vi "Get Targets.vi"(7 "Load Stored Targets?(T)":bool=TRUE, 8 "error in (no error)":errorcluster, 11 "Dependency Source in":refnum<class "Dependency Source.lvclass">) -> (0 "error out":errorcluster, 1 "Success?":bool, 2 "External Targets":T3, 3 "Internal Targets":T2, 4 "Unhandled Targets":T1, 5 "Valid Dependency Source?":bool)   [LabVIEW 2019, in "Project.Dependencies Finder.lvlib" / "Dependency Source.lvclass"]
doc: "Get internal and external targets for the dependency source."
uses:
  Dependency Source.lvclass
  Ctl/Ctl_External Target Element.ctl
  Ctl/Ctl_Internal Target Element.ctl
  Ctl/Ctl_Dependency Element.ctl
  Dependency Source.lvclass/Dependency Source.ctl
  Project.Dependencies Finder.lvlib
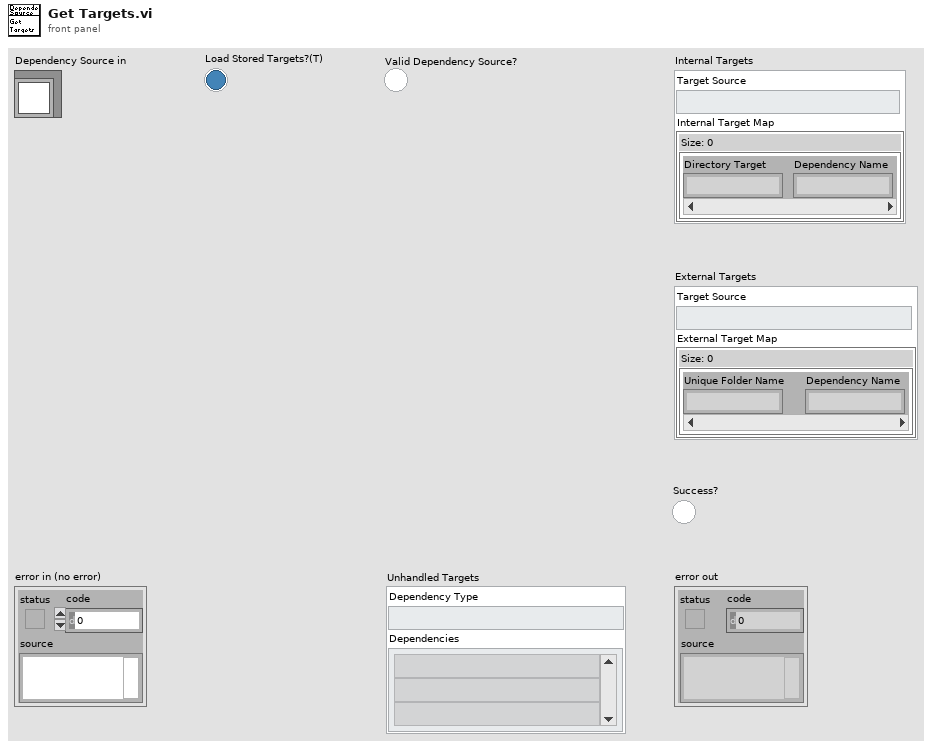
[diagram p1: front panel]
types:
  T1 = typedef "Project.Dependencies Finder.lvlib/Ctl_Dependency Element.ctl" = cluster{"Dependency Type":string, "Dependencies":string[]}
  T2 = typedef "Project.Dependencies Finder.lvlib/Ctl_Internal Target Element.ctl" = cluster{"Target Source":string, "Internal Target Map":map{string, string}}
  T3 = typedef "Project.Dependencies Finder.lvlib/Ctl_External Target Element.ctl" = cluster{"Target Source":string, "External Target Map":map{string, string}}
  T4 = typedef "Project.Dependencies Finder.lvlib/Ctl_Progress Queue.ctl" = refnum<queue>
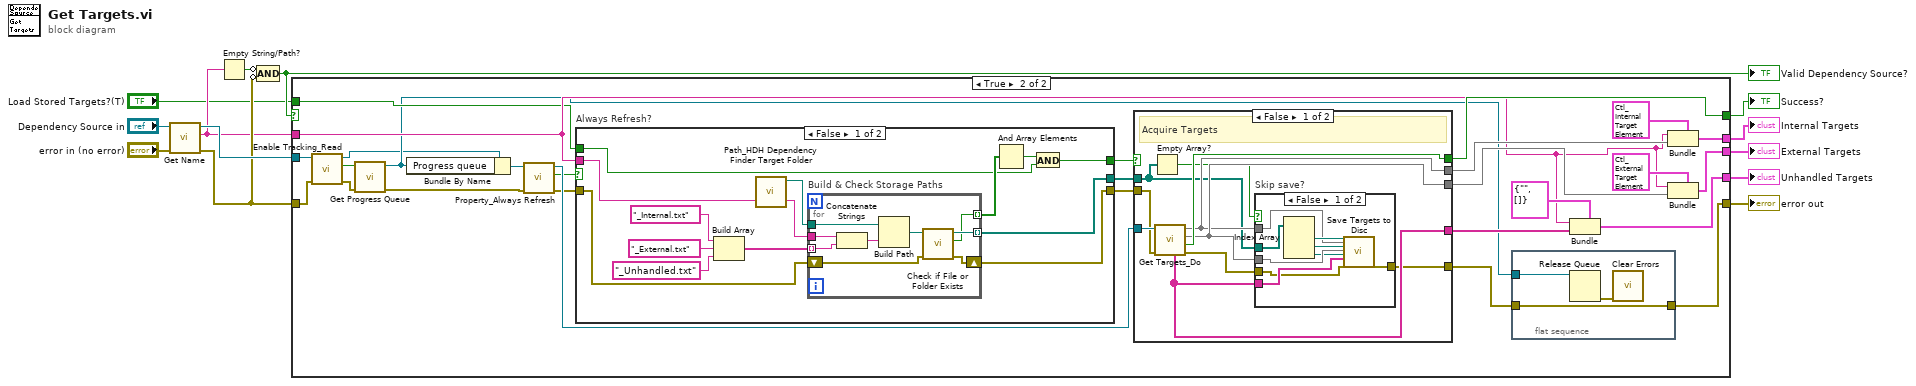
[diagram p0: block diagram]
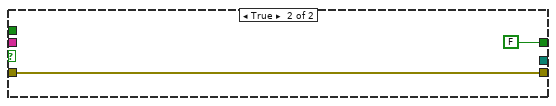
[diagram p3: hidden frame]
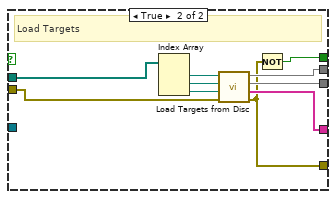
[diagram p5: hidden frame]
diagram:
  n1 = call-dynamic "Get Name.vi"("error in (no error)"="error in (no error)", "Dependency Source in"="Dependency Source in") -> ("error out"=w8:errorcluster, "Dependency Source Name"=w6:string, "Dependency Source out"=w11:refnum<class "Dependency Source.lvclass">)  [unwired: 7 in]
  n2 = Empty String/Path?(string/path=w6) -> (empty?=w9:bool)
  n3 = Compound Arithmetic op=AND(invert w9, invert w8) -> (w7:bool)
  "Valid Dependency Source?" <- w7
  n4 = case shown="True" w7 {
    selector: w7 -> [w14 _]
    tunnel: [w15 w27] -> w13
    tunnel: w11 -> [_ w23]
    tunnel: w8 -> [w15 w25]
    tunnel: w6 -> [_ w33]
    tunnel: [w14 w41] -> w5
    tunnel: [_ w40] -> w4
    tunnel: [_ w37] -> w3
    tunnel: [_ w34] -> w2
    tunnel: "Load Stored Targets?(T)" -> [_ w32]
    frame False {
    }
    frame True {
      n5 = call "Enable Tracking_Read.vi"("error in (no error)"=w25, "Dependency Source in"=w23) -> ("error out"=w26:errorcluster, "Enable Tracking?"=w22:bool, "Dependency Source out"=w24:refnum<class "Dependency Source.lvclass">)  [unwired: 7 in]
      n6 = call "Get Progress Queue.vi"("error in"=w26, "Enable Tracking?"=w22) -> ("error out"=w18:errorcluster, "Progress queue"=w29:T4)  [unwired: 8 in]
      n7 = Bundle By Name(cluster=w24, "Progress queue"=w29) -> (w20:refnum<class "Dependency Source.lvclass">)
      n8 = call-dynamic "Property_Always Refresh.vi"("error in (no error)"=w18, "Dependency Source in"=w20) -> ("error out"=w17:errorcluster, "Always Refresh Targets?"=w16:bool, "Dependency Source out"=w19:refnum<class "Dependency Source.lvclass">)  [unwired: 7 in]
      n9 = case "Always Refresh?" shown="False" w16 {
        tunnel: w33 -> [w56 _]
        tunnel: w32 -> [w48 _]
        tunnel: [w47 FALSE] -> w31
        tunnel: [w46 _] -> w30
        tunnel: [w45 w67] -> w21
        tunnel: w17 -> [w44 w67]
        frame False {
          n10 = Build Array("_Internal.txt" ("string"), "_External.txt" ("string"), "_Unhandled.txt" ("string")) -> (w51:string[])
          n11 = call "Path_HDH Dependency Finder Target Folder.vi"() -> ("HDH\\VIPM path"=w55:path)  [unwired: 10 in, 1 out]
          n12 = for "Build & Check Storage Paths" {
            tunnel: w56 -> [w65]
            tunnel: w55 -> [w64]
            tunnel: w51 -> [w59] mode=indexing
            tunnel: [w62] -> w46 mode=indexing
            tunnel: [w61] -> w50 mode=indexing
            shift-right: [w57] -> w45
            shift-left: w44 -> [w60]
            n13 = Concatenate Strings(w65, w59) -> (w58:string)
            n14 = Build Path(base path=w64, name or relative path=w58) -> (appended path=w63:path)
            n15 = call <vilib>:"Check if File or Folder Exists.vi"("error in (no error)"=w60, "path"=w63) -> ("error out"=w57:errorcluster, "file or folder exists?"=w61:bool, "dup path"=w62:path)  [unwired: 7 in]
          }
          n16 = And Array Elements(Boolean array=w50) -> (logical AND=w49:bool)
          n17 = And(x=w49, y=w48) -> (x .and. y?=w47:bool)
        }
        frame True {
        }
      }
      n18 = case shown="False" w31 {
        tunnel: [w73 w92] -> w28
        tunnel: w19 -> [w80 _]
        tunnel: [w76 w95] -> w42
        tunnel: [w79 w91] -> w41
        tunnel: [w77 w94] -> w38
        tunnel: [w75 w93] -> w35
        tunnel: w21 -> [w78 w96]
        tunnel: w30 -> [w72 w100]
        frame False {
          # "Acquire Targets"
          n19 = Empty Array?(array=w72) -> (empty?=w71:bool)
          n20 = call-dynamic "Get Targets_Do.vi"("error in (no error)"=w78, "Dependency Source in"=w80) -> ("error out"=w74:errorcluster, "Success?"=w79:bool, "External Target Map"=w77:map{string, string}, "Internal Target Map"=w76:map{string, string}, "Unhandled Targets"=w75:string[])  [unwired: 5 in]
          n21 = case "Skip save?" shown="False" w71 {
            tunnel: w72 -> [w89 _]
            tunnel: w77 -> [w87 _]
            tunnel: w76 -> [w86 _]
            tunnel: w75 -> [w84 _]
            tunnel: w74 -> [w82 w90]
            tunnel: [w81 w90] -> w73
            frame False {
              # "Save"
              n22 = Index Array(array=w89) -> (element #1=w88:path, element #2=w85:path, element #3=w83:path)  [unwired: 3 in]
              n23 = call "Save Targets to Disc.vi"("Internal Path"=w88, "Internal Target Map"=w86, "External Path"=w85, "External Target Map"=w87, "Unhandled Path"=w83, "Unhandled Dependencies"=w84, "error in (no error)"=w82) -> ("error out"=w81:errorcluster)  [unwired: 20 in]
            }
            frame True {
              # "Skip save"
            }
          }
        }
        frame True {
          # "Load Targets"
          n24 = Index Array(array=w100) -> (element #1=w99:path, element #2=w98:path, element #3=w97:path)  [unwired: 3 in]
          n25 = call "Load Targets from Disc.vi"("error in (no error)"=w96, "Unhandled Path"=w97, "External Path"=w98, "Internal Path"=w99) -> ("error out"=w92:errorcluster, "Unhandled Dependencies"=w93:string[], "External Target Map"=w94:map{string, string}, "Internal Target Map"=w95:map{string, string})  [unwired: 4 in]
          n26 = Not(x=w92) -> (.not. x?=w91:bool)
        }
      }
      n27 = flat-sequence {
        tunnel: w28 -> [w69]
        tunnel: w29 -> [w70]
        tunnel: [w69] -> w27
        frame #0 {
          n28 = Release Queue(queue=w70) -> (error out=w68:errorcluster)  [unwired: 2 in, 2 out]
          n29 = call <vilib>:"Clear Errors.vi"("error in (no error)"=w68) -> ()  [unwired: 5 in, 2 out]
        }
      }
      n30 = Bundle(cluster=T1 {"Dependency Type"="", "Dependencies"=[]} ("External Target Element"), "Dependency Type"=w33, "Dependencies"=w35) -> (w34:T1)
      n31 = Bundle(cluster=T2 {"Target Source"="", "Internal Target Map"={}} ("Internal Targets"), "Target Source"=w33, "Internal Target Map"=w42) -> (w40:T2)
      n32 = Bundle(cluster=T3 {"Target Source"="", "External Target Map"={}} ("External Targets"), "Target Source"=w33, "External Target Map"=w38) -> (w37:T3)
    }
  }
  "error out" <- w13
  "Internal Targets" <- w4
  "External Targets" <- w3
  "Success?" <- w5
  "Unhandled Targets" <- w2
